vi "PH_PPPA_PowerUnit.set i Attr.vi"(0 "i ref in":refnum<vi>, 5 "error in":errorcluster) -> (14 "i ref out":refnum<vi>, 17 "i Attribute":T1={"GUI Refs"={"Ignitron"=refnum, "Rossrelais"=refnum, "Set Voltage"=refnum, "PSU"=refnum, "EOC"=refnum, "Trigger"=refnum}, "Ignitron"={"State Device"=0, "linked?"=FALSE}, "PSU"={"lower limit [V]"=0.0, "upper limit [V]"=0.0, "Voltage set"=FALSE, "State Device"=0, "linked?"=FALSE}, "Dump Ross Relais"={"State Device"=0, "linked?"=FALSE}, "Trigger"={"State Device"=0, "linked?"=FALSE}, "Timing Settings"={"Prdc Fast?"=FALSE, "Default Value Periodic Interval"=0, "Mercury on since"=30.0, "Warm up Time Mercury [s]"=9999.0}, "Set Voltage [V]"=0.0, "19er Ignitionbox"="N/A"} {"Trigger"."State Device" items=["no info", "off/false/out", "on/true/in", "Failure", "Alarm", "Status 1", "Status 2", "Status 3"]; "Dump Ross Relais"."State Device" items=["no info", "off/false/out", "on/true/in", "Failure", "Alarm", "Status 1", "Status 2", "Status 3"]; "PSU"."State Device" items=["no info", "off/false/out", "on/true/in", "Failure", "Alarm", "Status 1", "Status 2", "Status 3"]; "Ignitron"."State Device" items=["no info", "off/false/out", "on/true/in", "Failure", "Alarm", "Status 1", "Status 2", "Status 3"]}, 19 "error out":errorcluster)   [LabVIEW 2014, in "PH_PPPA_PowerUnit.lvlib"]
doc: "In this VI the related instances which are not set in Read DB are set and written to own attributes."
uses:
  PH_PPPA_PowerUnit.lvlib
  PH_PPPA_PowerUnit.i attribute.ctl
  PH_PP_Common/PH_PP_Common.Ignitron Attributes.ctl
  PH_StatusHandler/PH_StatusHandler.Status.ctl
  PH_PP_Common/PH_PP_Common.PSU Attributes.ctl
  PH_PP_Common/PH_PP_Common.Ross Relais Attributes.ctl
  CSCore/BaseProcess/BaseProcess.lvlib
  PH_StatusHandler/PH_StatusHandler.lvlib
  PH_PP_Common/PH_PP_Common.lvlib
  PH_PowerUnit_BaseClass/PH_PowerUnit_BaseClass.lvlib
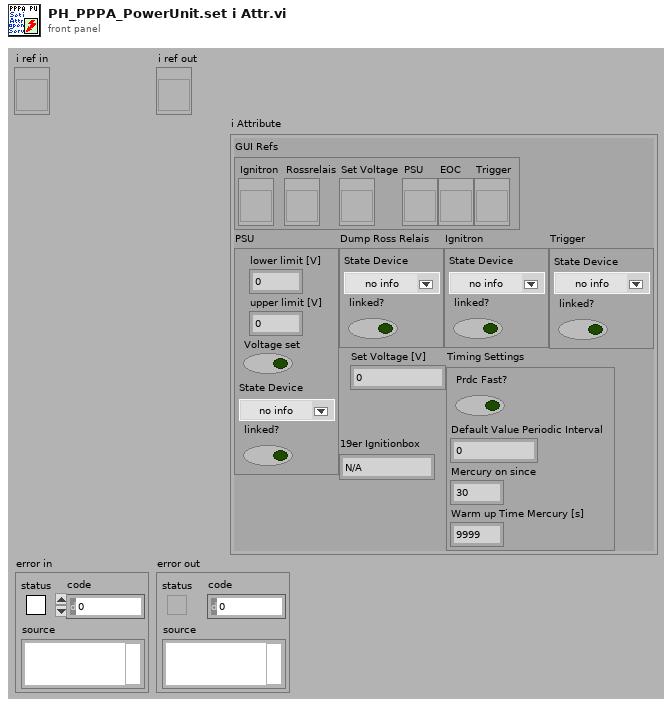
[diagram p1: front panel]
types:
  T1 = typedef "PH_PPPA_PowerUnit.lvlib/PH_PPPA_PowerUnit.i attribute.ctl" = cluster{"GUI Refs":cluster{"Ignitron":refnum<vi>, "Rossrelais":refnum<vi>, "Set Voltage":refnum<vi>, "PSU":refnum<vi>, "EOC":refnum<vi>, "Trigger":refnum<vi>}, "Ignitron":T2, "PSU":T4, "Dump Ross Relais":T5, "Trigger":cluster{"State Device":T3, "linked?":bool}, "Timing Settings":cluster{"Prdc Fast?":bool, "Default Value Periodic Interval":i32, "Mercury on since":dbl, "Warm up Time Mercury [s]":dbl}, "Set Voltage [V]":dbl, "19er Ignitionbox":string}
  T2 = typedef "PH_PP_Common.lvlib/PH_PP_Common.Ignitron Attributes.ctl" = cluster{"State Device":T3, "linked?":bool}
  T3 = typedef "PH_StatusHandler.lvlib/PH_StatusHandler.Status.ctl" = i16
  T4 = typedef "PH_PP_Common.lvlib/PH_PP_Common.PSU Attributes.ctl" = cluster{"lower limit [V]":dbl, "upper limit [V]":dbl, "Voltage set":bool, "State Device":T3, "linked?":bool}
  T5 = typedef "PH_PP_Common.lvlib/PH_PP_Common.Ross Relais Attributes.ctl" = cluster{"State Device":T3, "linked?":bool}
  T6 = typedef "PH_PowerUnit_BaseClass.lvlib/PH_PowerUnit_BaseClass.i attribute.ctl" = cluster{"Constructor finished":bool, "PU":cluster{"In use":bool, "Service ID in use":i32, "GUI Ref":refnum<vi>}, "Enabling":cluster{"State":T7, "GUI Ref":refnum<vi>}, "Timing":cluster{"Last Shot":dbl, "Time between Shots [Sec]":dbl, "Waiting Time over?":bool, "Service ID Waiting Time":i32, "GUI Ref":refnum<vi>, "Instance":cluster{"Status":T3, "linked?":bool, "GUI Ref":refnum<vi>}}, "Sequencer":cluster{"SM State":string, "GUI Ref":refnum<vi>, "linked":bool}, "Subscribed Trendmssgs":cluster{"Tagname":string, "Status":T3, "linked?":bool, "Shot Condition":T3, "GUI Ref":refnum<vi>}[], "PP PU":T8, "Default Voltage (V)":dbl, "GUI Refs":T9, "PSDB data":cluster{"Shot Voltage [V]":dbl, "State TO SM":T10, "Write 2 early":bool}, "State TO SM":T10}
  T7 = typedef "PH_SystemInformation.lvlib/PH_SystemInformationEnabling State.ctl" = i32
  T8 = typedef "PH_PP_Common.lvlib/PH_PP_Common.PUs.ctl" = enum16{"no Info", "PA-19mm-1", "PA-19mm-2", "PA-45mm-PILC", "PA-45mm-MAIN", "MA-PU-1", "MA-PU-2", "MA-PU-3", "MA-PU-4", "MA-PU-5", "MA-PU-6", "MA-FR", "MA-PILC", "PA-45mm-DP"}
  T9 = typedef "PH_PowerUnit_BaseClass.lvlib/PH_PowerUnit_BaseClass.GUI Refs.ctl" = cluster{"Delete Inst":refnum<vi>, "State TO SM":refnum<vi>, "State SM":refnum<vi>, "Fire":refnum<vi>}
  T10 = typedef "PH_PowerUnit_BaseClass.lvlib/PH_PowerUnit_BaseClass.SM States.ctl" = enum16{".", "Stand by", "Switch PU on", "Configure", "Set Default Voltage", "Set STANDBY", "Set READY", "Wait for Shot Cmd", "Open Dump Rods", "Open Ross Relais", "Close Ross Relais", "Switch PSU on", "Switch PSU off", "Charge", "Switch GD Channel on", "Close Dump Rods", "Rods-TO", "RR-TO", "PSU-TO", "Trigger-TO"}
  T11 = typedef "BaseProcess.lvlib/BaseProcess.i attribute.ctl" = cluster{"EventStatus":string, "EventError":i32, "PresetEvtWatchD":i32, "PresetPdcWatchD":i32, "EventTimeout":i32, "PeriodicInterval":i32, "Interface":string[], "Address":string[], "Special":string[], "PeriodicError":i32, "PeriodicStatus":string, "SuperProc":string, "Descriptors":T12[], "CaseRef":refnum<vi>, "PdcRef":refnum<vi>, "Thread Ref":refnum<vi>, "eventErrorID":i32, "eventStatusID":i32, "periodicErrorID":i32, "periodicStatusID":i32, "pdcCtrID":i32}
  T12 = typedef "BaseProcess.lvlib/BaseProcess.descriptor definition.ctl" = cluster{"selector":string, "descriptor":T13}
  T13 = typedef "BaseProcess.lvlib/BaseProcess.descriptor string definition.ctl" = string
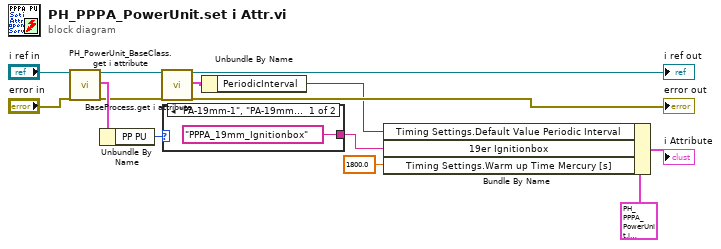
[diagram p0: block diagram]
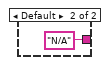
[diagram p2: hidden frame]
diagram:
  n1 = call "PH_PowerUnit_BaseClass.get i attribute.vi"("i ref in"="i ref in", "error in (no error)"="error in") -> ("i ref out"=w8:refnum<vi>, "i attribute"=w4:T6, "error out"=w1:errorcluster)  [unwired: 15 in]
  n2 = Unbundle By Name(w4) -> ("PP PU"=w3:T8)
  n3 = call "BaseProcess.get i attribute.vi"("i ref in"=w8, "error in (no error)"=w1) -> ("i ref out"=→"i ref out":refnum<vi>, "i attribute"=w7:T11, "error out"=→"error out":errorcluster)  [unwired: 15 in]
  n4 = case shown="\"PA-19mm-1\", \"PA-19mm-2\"" w3 {
    tunnel: ["PPPA_19mm_Ignitionbox" "N/A"] -> w9
    frame "PA-19mm-1", "PA-19mm-2" {
    }
    frame Default {
    }
  }
  n5 = Unbundle By Name(w7) -> ("PeriodicInterval"=w6:i32)
  n6 = Bundle By Name(cluster=T1 {"GUI Refs"={"Ignitron"=refnum, "Rossrelais"=refnum, "Set Voltage"=refnum, "PSU"=refnum, "EOC"=refnum, "Trigger"=refnum}, "Ignitron"={"State Device"=0, "linked?"=FALSE}, "PSU"={"lower limit [V]"=0.0, "upper limit [V]"=0.0, "Voltage set"=FALSE, "State Device"=0, "linked?"=FALSE}, "Dump Ross Relais"={"State Device"=0, "linked?"=FALSE}, "Trigger"={"State Device"=0, "linked?"=FALSE}, "Timing Settings"={"Prdc Fast?"=FALSE, "Default Value Periodic Interval"=0, "Mercury on since"=30.0, "Warm up Time Mercury [s]"=9999.0}, "Set Voltage [V]"=0.0, "19er Ignitionbox"="N/A"} ("i attribute"), "Timing Settings.Default Value Periodic Interval"=w6, "19er Ignitionbox"=w9, "Timing Settings.Warm up Time Mercury [s]"=1800.0) -> (→"i Attribute":T1)
